vi "Initialize RF Sessions From Pinmap.vi"(0 "TSM Context":T1, 5 "Fixture Or Cal":string, 11 "Error in":errorcluster) -> (4 "RF SubSystem Session Providers":refnum<class "RF Subsystem Session Provider.lvclass">[](array[class]), 15 "Error out":errorcluster)   [LabVIEW 2023, in "RFCalAndFixtureCharact.Common.lvlib"]
uses:
  RFCalAndFixtureCharact.Common.lvlib
  <vilib>/NI_TestStand_SemiconductorModule/NI_TestStand_Semiconductor_Module.lvlibp/PinMap/General/SemiconductorModuleContext.ctl
  RF Subsystem Session Provider/RF Subsystem Session Provider.lvclass
  <vilib>/NI_TestStand_SemiconductorModule/NI_TestStand_Semiconductor_Module.lvlibp
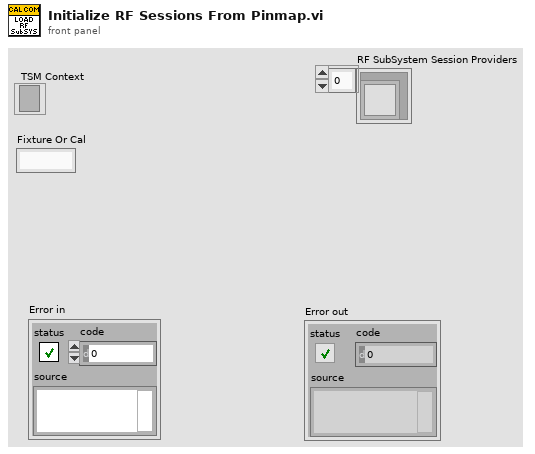
[diagram p1: front panel]
types:
  T1 = typedef "NI_TestStand_Semiconductor_Module.lvlibp/SemiconductorModuleContext.ctl" = refnum<k7>
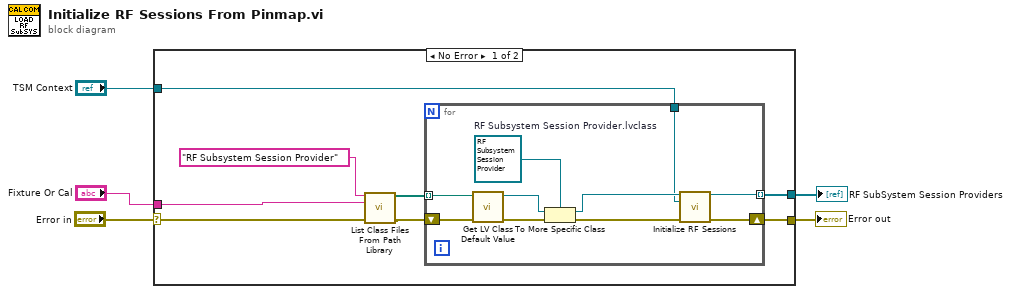
[diagram p0: block diagram]
diagram:
  n1 = case shown="No Error" "Error in" {
    selector: "Error in" -> [w10 w24]
    tunnel: [w13 w24] -> w5
    tunnel: "TSM Context" -> [w12 _]
    tunnel: [w11 _] -> w2
    tunnel: "Fixture Or Cal" -> [w6 _]
    frame No Error {
      n2 = call "List Class Files From Path Library.vi"("Specified Folder Name"="RF Subsystem Session Provider", "Fixture Or Cal"=w6, "Error in"=w10) -> ("Class Files"=w7:path[], "Error out"=w9:errorcluster)  [unwired: 11 in]
      n3 = for {
        shift-right: [w16] -> w13
        shift-left: w9 -> [w23]
        tunnel: w7 -> [w22] mode=indexing
        tunnel: w12 -> [w15]
        tunnel: [w14] -> w11 mode=indexing
        w20 = refnum<class "RF Subsystem Session Provider.lvclass"> refnum  # RF Subsystem Session Provider.lvclass
        n4 = call <vilib>:"Get LV Class Default Value.vi"("error in (no error)"=w23, "class path"=w22) -> ("error out"=w21:errorcluster, "object"=w19:refnum<class>)  [unwired: 8 in]
        n5 = To More Specific Class(target class=w20, reference=w19, error in=w21) -> (specific class reference=w18:refnum<class "RF Subsystem Session Provider.lvclass">, error out=w17:errorcluster)
        n6 = call-dynamic "Initialize RF Sessions.vi"("RF Subsystem Session Provider in"=w18, "TSM Context"=w15, "error in"=w17) -> ("RF Subsystem Session Provider out"=w14:refnum<class "RF Subsystem Session Provider.lvclass">, "error out"=w16:errorcluster)  [unwired: 11 in]
      }
    }
    frame Error {
    }
  }
  "Error out" <- w5
  "RF SubSystem Session Providers" <- w2
